vi "calculate massflow.vi"(8 "Temp (C)":dbl, 9 "Differential pressure (bar)":dbl, 10 "Upstream static gauge pressure (Pa)":dbl, 11 "Ambient pressure (Pa)":dbl) -> (1 "Flowrate":dbl caption="V-Cone Mass Flowrate (Kg/s)", 3 "Volume Flowrate (m3/s)":dbl)   [LabVIEW 2018]
uses:
  Chris VIs/V-cone/V-Cone CompressorRig.vi
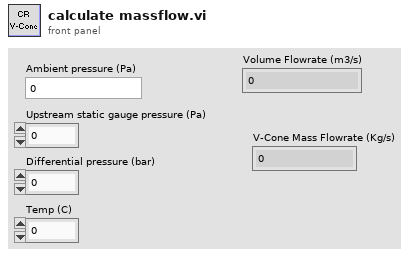
[diagram p1: front panel]
types:
  T1 = cluster{"delta P (mBar)":dbl, "T (K)":dbl, "High (bar)":dbl}
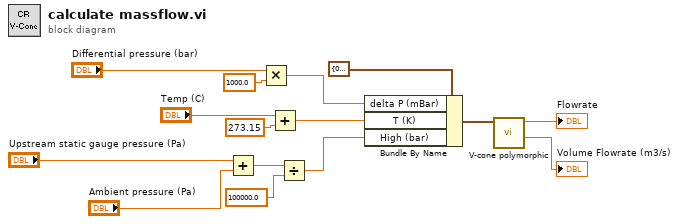
[diagram p0: block diagram]
diagram:
  n1 = Add(x="Upstream static gauge pressure (Pa)", y="Ambient pressure (Pa)") -> (x+y=w10:dbl)
  n2 = Multiply(x="Differential pressure (bar)", y=1000.0) -> (x*y=w2:dbl)
  n3 = Add(x="Temp (C)", y=273.15) -> (x+y=w8:dbl)
  n4 = Divide(x=w10, y=100000.0 ("x")) -> (x/y=w9:dbl)
  n5 = Bundle By Name(cluster=T1 {"delta P (mBar)"=0.0, "T (K)"=0.0, "High (bar)"=0.0} ("Measurements"), "delta P (mBar)"=w2, "T (K)"=w8, "High (bar)"=w9) -> (w5:T1)
  n6 = call-poly "V-cone polymorphic.vi"("Measurements"=w5) -> ("Volume Flowrate (m3/s)"=→"Volume Flowrate (m3/s)":dbl, "Mass Flowrate (Kg/s)"=→"Flowrate":dbl)  [unwired: 9 in]
